vi "Get Temperature.vi"(7 "VISA resource":refnum<visa-resource-name>, 8 "error in (no error)":errorcluster, 9 "Name":string, 10 "Data":T1={"Record heater"=FALSE, "Record RAW"=FALSE, "Set point"=0.0, "Heater range"=0.0, "Approach"=enum."Instant", "Ramp rate, K/min"=1.0, "Record Channels"=[], "Settling time "=60.0, "Settling range"=0.1, "P"=0.0, "I"=0.0, "D"=0.0, "Temperature Control"=FALSE}, 11 "Cryo-Con in":refnum<class "Cryo-Con.lvclass">) -> (0 "error out":errorcluster, 1 "Channel data":dbl[](array[numeric]), 2 "Channel names":string[](array[string]), 3 "Cryo-Con out":refnum<class "Cryo-Con.lvclass">, 4 "Controled temperature":dbl, 5 "VISA resource out":refnum<visa-resource-name>)   [LabVIEW 2015, in "Cryo-Con.lvclass"]
uses:
  Cryo-Con.lvclass
  Temperarture Controller/T controller parameters.ctl
  Instruments/Neocera/Neocera Set Point Aproach.ctl
panel:
  # "Temperature Monitor"
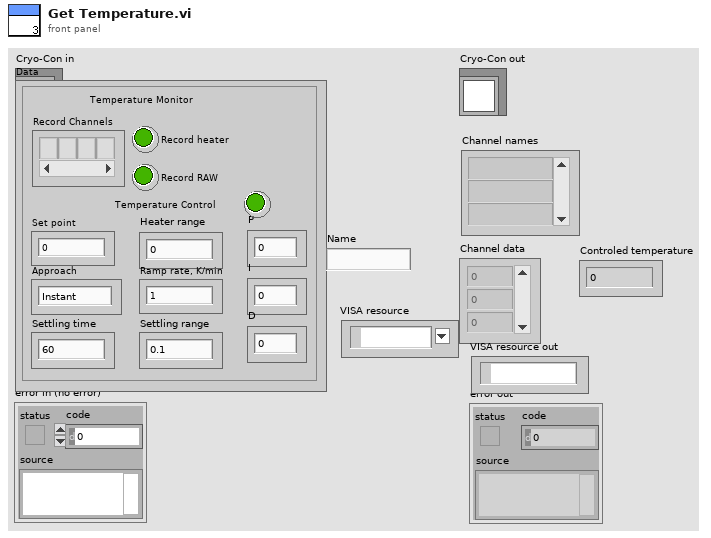
[diagram p1: front panel]
types:
  T1 = typedef "T controller parameters.ctl" = cluster{"Record heater":bool, "Record RAW":bool, "Set point":dbl, "Heater range":dbl, "Approach":T2, "Ramp rate, K/min":dbl, "Record Channels":string[], "Settling time ":dbl, "Settling range":dbl, "P":dbl, "I":dbl, "D":dbl, "Temperature Control":bool}
  T2 = typedef "Neocera Set Point Aproach.ctl" = enum16{"Instant", "Ramp"}
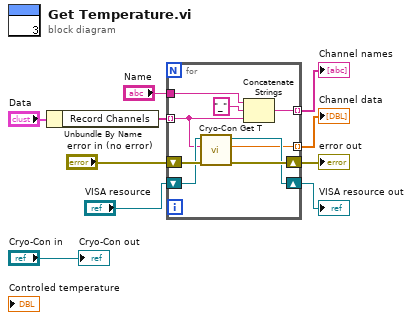
[diagram p0: block diagram]
diagram:
  n1 = Unbundle By Name("Data") -> ("Record Channels"=w10:string[])
  n2 = for {
    tunnel: [w11] -> w8 mode=indexing
    shift-right: [w14] -> w6
    shift-left: "VISA resource" -> [w13]
    shift-right: [w15] -> w7
    shift-left: "error in (no error)" -> [w16]
    tunnel: w10 -> [w12] mode=indexing
    tunnel: "Name" -> [w19]
    tunnel: [w17] -> w9 mode=indexing
    n3 = call "Cryo-Con Get T.vi"("error in (no error)"=w16, "Channel"=w12, "VISA Resource Name"=w13) -> ("error out"=w15:errorcluster, "Temperature"=w11:dbl, "VISA Resource Name Out"=w14:refnum<visa-resource-name>)  [unwired: 5 in, 1 out]
    n4 = Concatenate Strings(w19, "_" ("string"), w12) -> (w17:string)
  }
  "error out" <- w7
  "VISA resource out" <- w6
  "Channel data" <- w8
  "Channel names" <- w9
  "Cryo-Con out" <- "Cryo-Con in"
